vi "Curr2Torq.vi"(1 "Current":dbl[](array[numeric])) -> (0 "Torque":dbl[](array[numeric]))   [LabVIEW 2014]
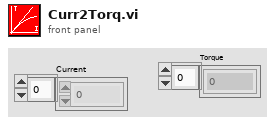
[diagram p1: front panel]
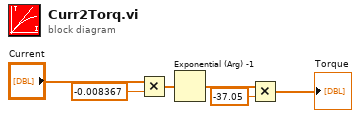
[diagram p0: block diagram]
diagram:
  n1 = Multiply(x="Current", y=-0.008367) -> (x*y=w5:dbl[])
  n2 = Exponential (Arg) -1(1:w5) -> (0:w4:dbl[])
  n3 = Multiply(x=w4, y=-37.05) -> (x*y=→"Torque":dbl[])
